vi "VI-Hacker.vi"   [LabVIEW 2021]
doc: "Unlocks the active password protected VI."
uses:
  _VI-Hacker/VI-Hacker.lvlib
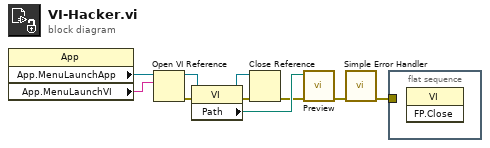
[diagram p0: block diagram]
diagram:
  n1 = property class="App"() -> ("App.MenuLaunchApp"=w3:refnum<vi>, "App.MenuLaunchVI"=w2:string)  [unwired: 2 in, 2 out]
  n2 = Open VI Reference(application reference (local)=w3, vi path=w2) -> (vi reference=w6:refnum<vi>, error out=w7:errorcluster)  [unwired: 4 in]
  n3 = property class="VI"(reference=w6, error in=w7) -> (reference out=w4:refnum<vi>, error out=w8:errorcluster, "Path"=w10:path)
  n4 = Close Reference(reference=w4, error in (no error)=w8) -> (error out=w5:errorcluster)
  n5 = call "Preview.vi"("error in (no error)"=w5, "Password Protected VI Path"=w10) -> ("error out"=w9:errorcluster)  [unwired: 9 in]
  n6 = call <vilib>:"Simple Error Handler.vi"("error in (no error)"=w9) -> ("error out"=w1:errorcluster)  [unwired: 4 in, 4 out]
  n7 = flat-sequence {
    tunnel: w1 -> [_]
    frame #0 {
      n8 = invoke class="VI" method="FP.Close"() -> ()  [unwired: 3 in, 3 out]
    }
  }
